vi "Microphone Board Test.vi"(5 "Test Config":T1={"Chopper RPM"=140, "IR Power"=5, "Conc Tolerance"=0.0, "Gas Stable Time"=0, "A-D Settle"=0, "Samples"=0, "Filter Time"=0, "Gas Mixtures"=[], "Filter Sequences"=[], "Functional Test"={"Mic Test ON ADC Max"=0.0, "Mic Test ON ADC Min"=0.0, "Mic Test OFF ADC Max"=0.0, "Mic Test OFF ADC Min"=0.0, "Mic Test IC ADC Max"=0.0, "Mic Test IC ADC Min"=0.0, "IR Emitter ON ADC Max"=0.0, "IR Emitter ON ADC Min"=0.0, "IR Emitter OFF ADC Max"=0.0, "IR Emitter OFF ADC Min"=0.0}, "Initial Flow Rate"=0.0, "Max Flow Rate"=0.0} {"Gas Mixtures"."ADC Gains" items=["0"=0, "3"=3, "4"=4, "5"=5, "6"=6, "7"=7]; "Conc Tolerance" min=0.0 max=100.0 step=1.0; "IR Power" min=2 max=5 step=1; "Chopper RPM" min=140 max=1000 step=1}, 8 "error in (no error)":errorcluster, 11 "Session Handle in":T6) -> (0 "error out":errorcluster, 1 "Failure Reason":string, 2 "Success?":bool, 3 "Session Handle out":T6 caption="Gas")   [LabVIEW 2015, in "PAS.lvclass"]
uses:
  PAS.lvclass
  Typedefs/Session Handle.ctl
  Tests/Controls/Test Config.ctl
  Tests/Controls/Gas Mixture.ctl
  Typedefs/ADC Gains.ctl
  Tests/Controls/Filter Sequence.ctl
  Tests/Controls/Functional Test.ctl
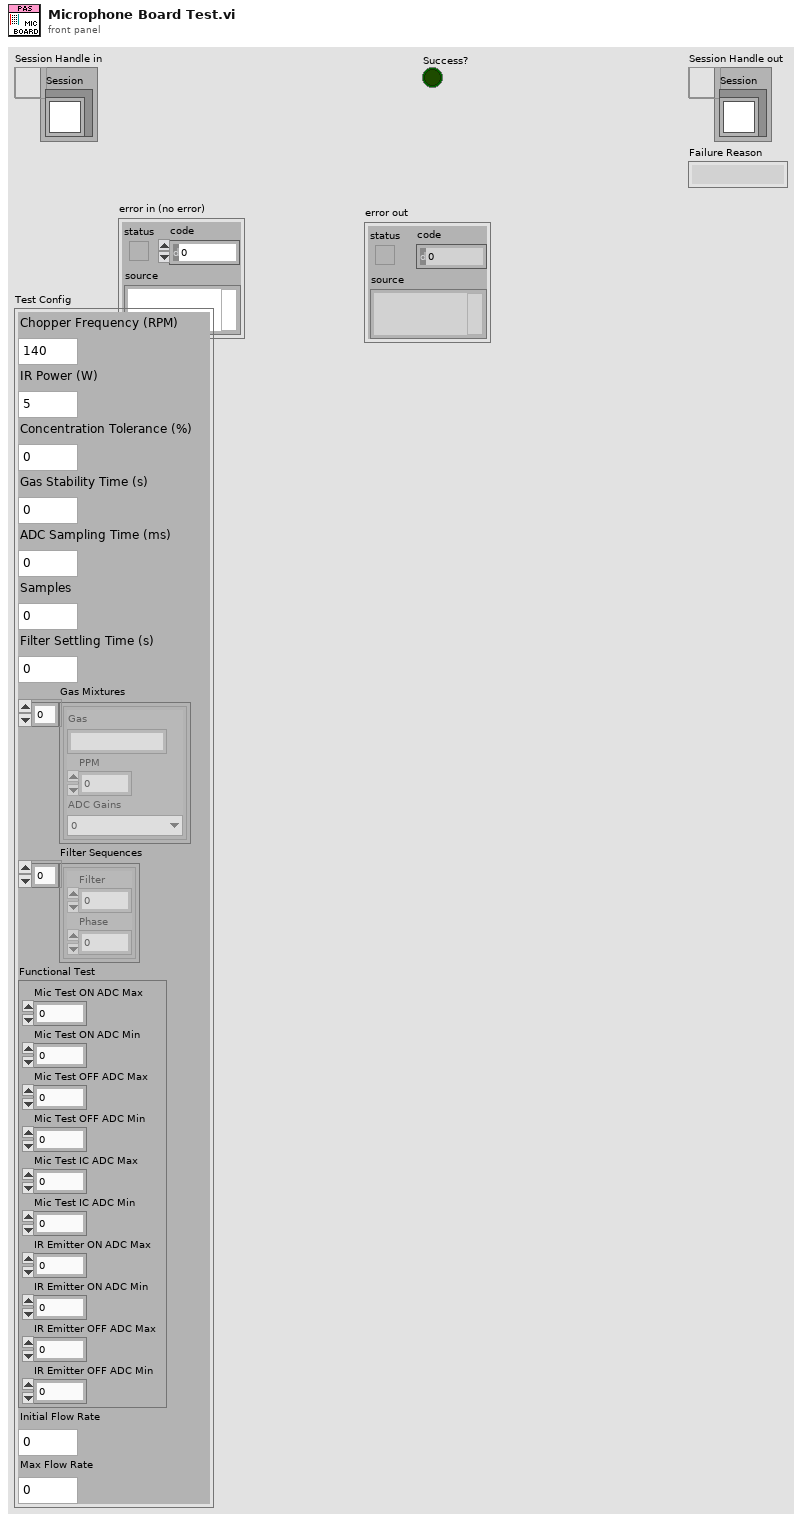
[diagram p1: front panel]
types:
  T1 = typedef "Test Config.ctl" = cluster{"Chopper RPM":u16, "IR Power":u8, "Conc Tolerance":dbl, "Gas Stable Time":u16, "A-D Settle":u16, "Samples":u16, "Filter Time":u16, "Gas Mixtures":T2[], "Filter Sequences":T4[], "Functional Test":T5, "Initial Flow Rate":sgl, "Max Flow Rate":sgl}
  T2 = typedef "Gas Mixture.ctl" = cluster{"Gas":string, "PPM":dbl, "ADC Gains":T3}
  T3 = typedef "PAS.lvclass/ADC Gains.ctl" = u16
  T4 = typedef "Filter Sequence.ctl" = cluster{"Filter":u8, "Phase":dbl}
  T5 = typedef "Functional Test.ctl" = cluster{"Mic Test ON ADC Max":dbl, "Mic Test ON ADC Min":dbl, "Mic Test OFF ADC Max":dbl, "Mic Test OFF ADC Min":dbl, "Mic Test IC ADC Max":dbl, "Mic Test IC ADC Min":dbl, "IR Emitter ON ADC Max":dbl, "IR Emitter ON ADC Min":dbl, "IR Emitter OFF ADC Max":dbl, "IR Emitter OFF ADC Min":dbl}
  T6 = typedef "PAS.lvclass/Session Handle.ctl" = refnum<data-value>
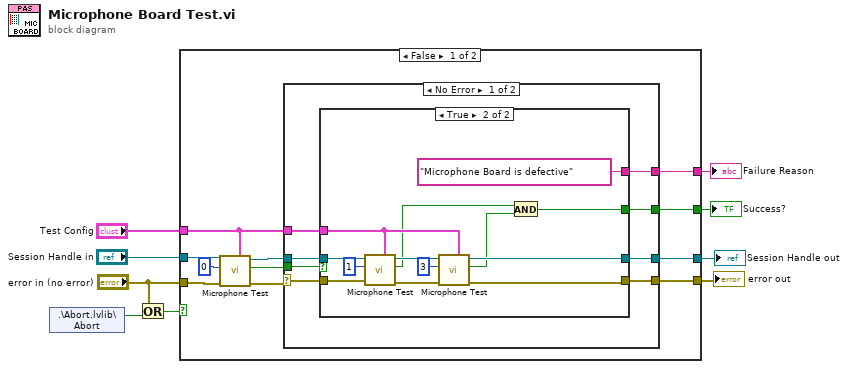
[diagram p0: block diagram]
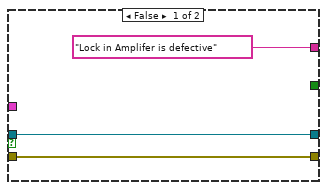
[diagram p2: hidden frame]
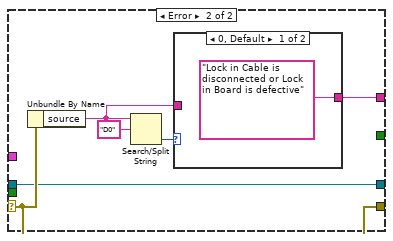
[diagram p3: hidden frame]
diagram:
  n1 = shared-variable ".\\Abort.lvlib\\Abort"() -> (w8:bool)  [unwired: 1 in, 1 out]
  n2 = Or(x="error in (no error)", y=w8) -> (x .or. y?=w9:bool)
  n3 = case shown="False" w9 {
    tunnel: "error in (no error)" -> [w20 w54]
    tunnel: "Session Handle in" -> [w19 w53]
    tunnel: "Test Config" -> [w10 _]
    tunnel: [w15 w54] -> w3
    tunnel: [w13 _] -> w5
    tunnel: [w12 w53] -> w4
    tunnel: [w11 _] -> w2
    frame False {
      n4 = call "Microphone Test.vi"("Test Config"=w10, "error in (no error)"=w20, "Mic Command"=u8 0, "Session Handle in"=w19) -> ("error out"=w17:errorcluster, "Success?"=w16:bool, "Session Handle out"=w14:T6)  [unwired: 4 in, 1 out]
      n5 = case shown="No Error" w17 {
        selector: w17 -> [w28 w46]
        tunnel: [w25 w47] -> w11
        tunnel: w16 -> [w27 _]
        tunnel: [w26 w46] -> w15
        tunnel: w14 -> [w24 w45]
        tunnel: w10 -> [w23 _]
        tunnel: [w22 _] -> w13
        tunnel: [w21 w45] -> w12
        frame No Error {
          n6 = case shown="True" w27 {
            tunnel: w28 -> [w31 w44]
            tunnel: [w31 w36] -> w26
            tunnel: ["Lock in Amplifer is defective" ("source") "Microphone Board is defective" ("source")] -> w25
            tunnel: w24 -> [w29 w43]
            tunnel: w23 -> [_ w39]
            tunnel: [w29 w37] -> w21
            tunnel: [_ w33] -> w22
            frame False {
            }
            frame True {
              n7 = call "Microphone Test.vi"("Test Config"=w39, "error in (no error)"=w44, "Mic Command"=u8 1, "Session Handle in"=w43) -> ("error out"=w41:errorcluster, "Success?"=w35:bool, "Session Handle out"=w40:T6)  [unwired: 4 in, 1 out]
              n8 = call "Microphone Test.vi"("Test Config"=w39, "error in (no error)"=w41, "Mic Command"=u8 3, "Session Handle in"=w40) -> ("error out"=w36:errorcluster, "Success?"=w34:bool, "Session Handle out"=w37:T6)  [unwired: 4 in, 1 out]
              n9 = And(x=w35, y=w34) -> (x .and. y?=w33:bool)
            }
          }
        }
        frame Error {
          n10 = Unbundle By Name(w46) -> ("source"=w48:string)
          n11 = Search/Split String(string=w48, search string/char (-)="D0") -> (offset of match=w49:i32)  [unwired: 1 in, 2 out]
          n12 = case shown="0, Default" w49 {
            tunnel: ["Lock in Cable is disconnected or Lock in Board is defective" ("source") w52] -> w47
            tunnel: w48 -> [_ w52]
            frame 0, Default {
            }
            frame -1 {
            }
          }
        }
      }
    }
    frame True {
    }
  }
  "error out" <- w3
  "Success?" <- w5
  "Session Handle out" <- w4
  "Failure Reason" <- w2
